vi "Data_Element_Retrieved.vi"(9 "文件名":string, 10 "路径":path=path "F:/report", 11 "Cluster67":T1) -> ()   [LabVIEW 2019]
uses:
  Cluster67.ctl
  <vilib>/Utility/NIReport.llb/Report Type.ctl
  <vilib>/addons/_office/word.llb/Word Find & Replace (str).vi
  <vilib>/Utility/NIReport.llb/NI_ReportGenerationCore.lvlib
  <vilib>/Utility/NIReport.llb/NI_report.lvclass
  <vilib>/addons/_office/NI_ReportGenerationToolkit.lvlib
  <vilib>/Utility/NIReport.llb/Word/NI_Word.lvclass
  TEST.lvclass
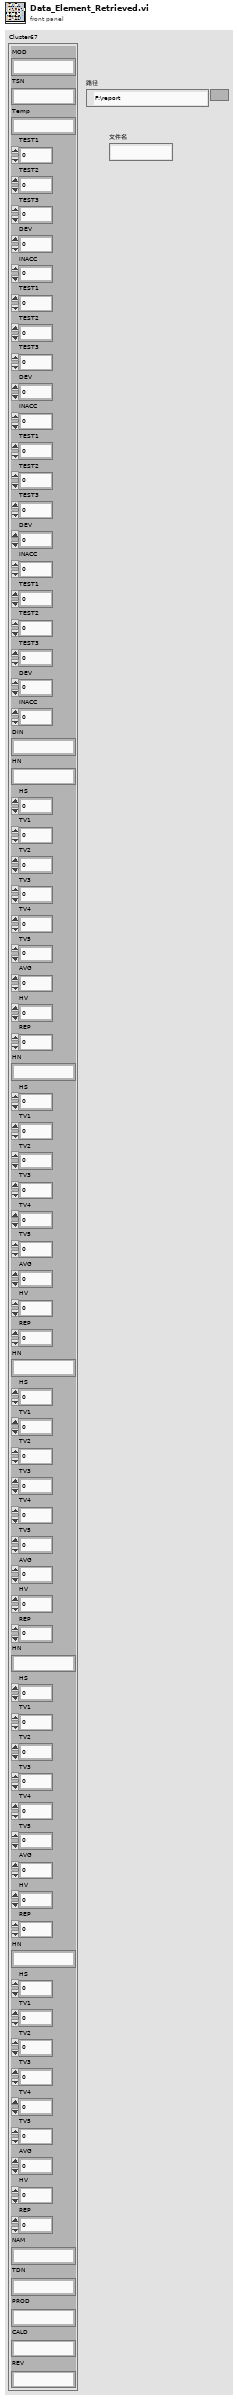
[diagram p1: front panel]
types:
  T1 = typedef "TEST.lvclass/Cluster67.ctl" = cluster{"MOD":string, "TSN":string, "Temp":string, "TEST1":sgl, "TEST2":sgl, "TEST3":sgl, "DEV":sgl, "INACC":sgl, "TEST1":sgl, "TEST2":sgl, "TEST3":sgl, "DEV":sgl, "INACC":sgl, "TEST1":sgl, "TEST2":sgl, "TEST3":sgl, "DEV":sgl, "INACC":sgl, "TEST1":sgl, "TEST2":sgl, "TEST3":sgl, "DEV":sgl, "INACC":sgl, "DIN":string, "HN":string, "HS":sgl, "TV1":sgl, "TV2":sgl, "TV3":sgl, "TV4":sgl, "TV5":sgl, "AVG":sgl, "HV":sgl, "REP":sgl, "HN":string, "HS":sgl, "TV1":sgl, "TV2":sgl, "TV3":sgl, "TV4":sgl, "TV5":sgl, "AVG":sgl, "HV":sgl, "REP":sgl, "HN":string, "HS":sgl, "TV1":sgl, "TV2":sgl, "TV3":sgl, "TV4":sgl, "TV5":sgl, "AVG":sgl, "HV":sgl, "REP":sgl, "HN":string, "HS":sgl, "TV1":sgl, "TV2":sgl, "TV3":sgl, "TV4":sgl, "TV5":sgl, "AVG":sgl, "HV":sgl, "REP":sgl, "HN":string, "HS":sgl, "TV1":sgl, "TV2":sgl, "TV3":sgl, "TV4":sgl, "TV5":sgl, "AVG":sgl, "HV":sgl, "REP":sgl, "NAM":string, "TDN":string, "PROD":string, "CALD":string, "REV":string}
  T2 = typedef "NI_ReportGenerationCore.lvlib/Report Type.ctl" = enum16{"HTML", "Word", "Excel"}
  T3 = enum16{"maximized", "minimized", "normal", "no change"}
  T4 = typedef "TEST.lvclass/Test_data.ctl" = cluster{"MODE":string, "TSN":string, "Temp":string, "Test_load_row1":T5, "Test_load_row2":T5, "Test_load_row3":T5, "Test_load_row4":T5, "DIN":string, "Hardness_test_row1":T6, "Hardness_test_row2":T6, "Hardness_test_row3":T6, "Hardness_test_row4":T6, "Hardness_test_row5":T6}
  T5 = typedef "TEST.lvclass/Test_load.ctl" = cluster{"TEST1":sgl, "TEST2":sgl, "TEST3":sgl, "DEV":sgl, "INACC":sgl}
  T6 = typedef "TEST.lvclass/Hardness_test.ctl" = cluster{"HN":string, "HS":sgl, "TV1":sgl, "TV2":sgl, "TV3":sgl, "TV4":sgl, "TV5":sgl, "AVG":sgl, "HV":sgl, "REP":sgl}
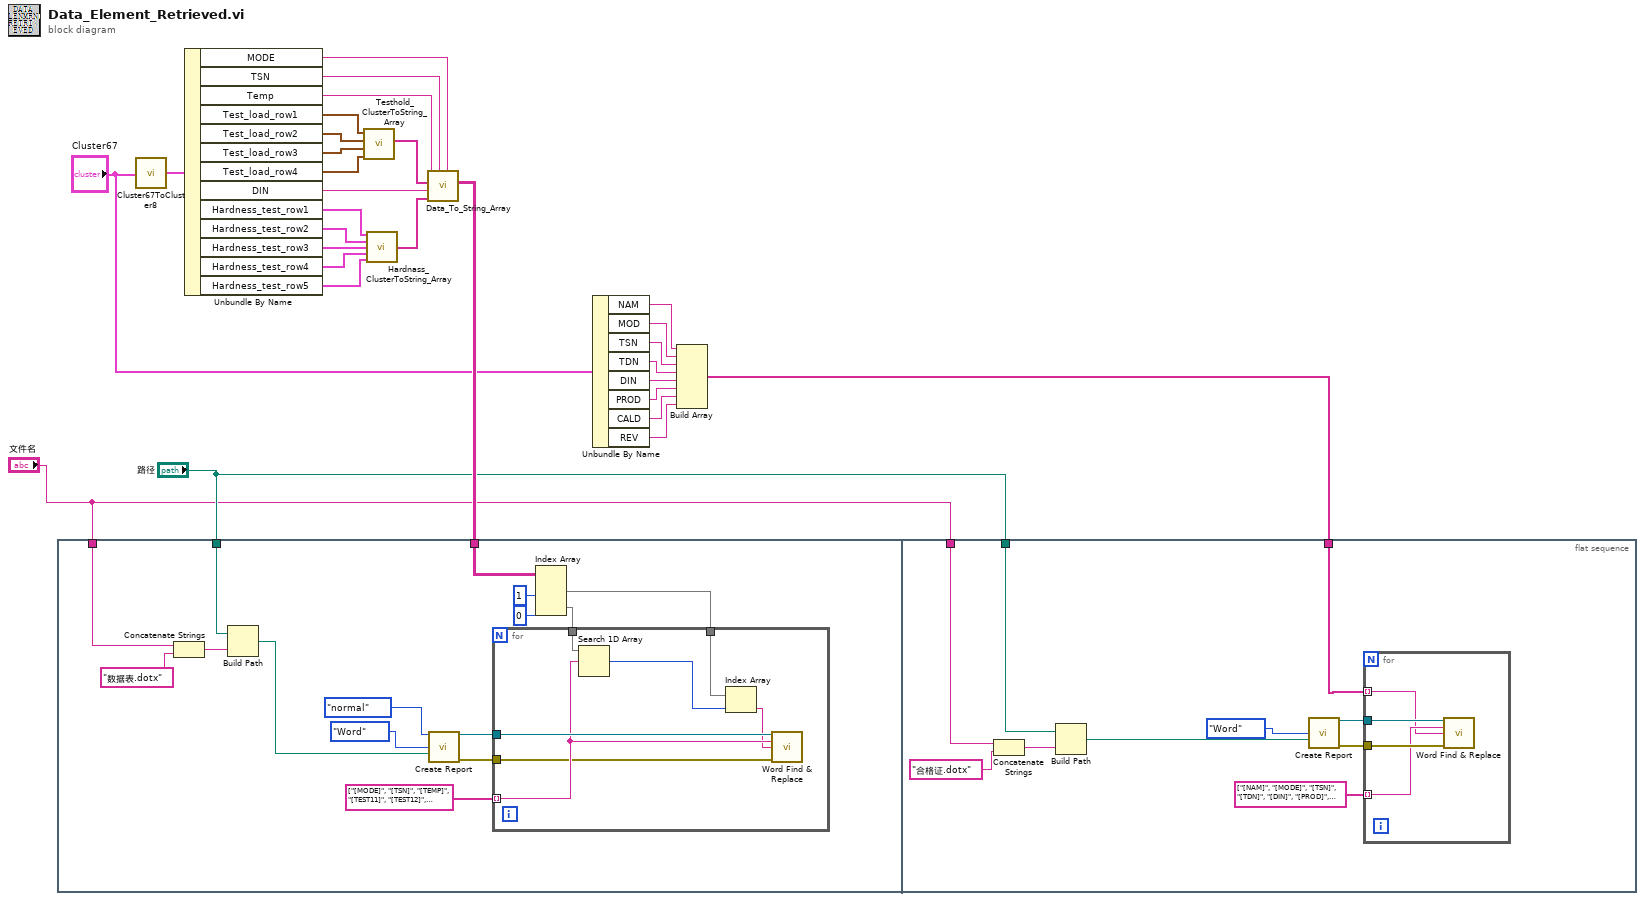
[diagram p0: block diagram]
diagram:
  n1 = flat-sequence {
    tunnel: w13 -> [w35]
    tunnel: "路径" -> [w39]
    tunnel: "文件名" -> [w36]
    tunnel: "路径" -> [w54]
    tunnel: "文件名" -> [w53]
    tunnel: w2 -> [w52]
    frame #0 {
      n2 = Concatenate Strings(w36, "数据表.dotx" ("字符串")) -> (w38:string)
      n3 = Build Path(base path=w39, name or relative path=w38) -> (appended path=w40:path)
      n4 = call <vilib>:"Create Report.vi"("window state (normal)"=T3."normal", "report type"=Report_Type."Word", "template (empty)"=w40) -> ("report out"=w42:refnum<class "NI_report.lvclass">, "error out"=w41:errorcluster)  [unwired: 11 in]
      n5 = Index Array(array=w35, index (col) #1=1 ("禁用的索引 (列)"), index (col) #2=0 ("索引 (列)")) -> (element #1=w31:string[], element #2=w32:string[])  [unwired: 2 in]
      n6 = for {
        tunnel: string[] ["[MODE]", "[TSN]", "[TEMP]", "[TEST11]", "[TEST12]", "[TEST13]", "[DEV1]", "[INACC1]", "[TEST21]", "[TEST22]", "[TEST23]", "[DEV2]", "[INACC2]", "[TEST31]", "[TEST32]", "[TEST33]", "[DEV3]", "[INACC3]", "[TEST41]", "[TEST42]", "[TEST43]", "[DEV4]", "[INACC4]", "[DIN]", "[HN1]", "[HS1]", "[TV11]", "[TV12]", "[TV13]", "[TV14]", "[TV15]", "[AVG1]", "[HV1]", "[REP1]", "[HN2]", "[HS2]", "[TV21]", "[TV22]", "[TV23]", "[TV24]", "[TV25]", "[AVG2]", "[HV2]", "[REP2]", "[HN3]", "[HS3]", "[TV31]", "[TV32]", "[TV33]", "[TV34]", "[TV35]", "[AVG3]", "[HV3]", "[REP3]", "[HN4]", "[HS4]", "[TV41]", "[TV42]", "[TV43]", "[TV44]", "[TV45]", "[AVG4]", "[HV4]", "[REP4]", "[HN5]", "[HS5]", "[TV51]", "[TV52]", "[TV53]", "[TV54]", "[TV55]", "[AVG5]", "[HV5]", "[REP5]"] ("待写入项") -> [w50] mode=indexing
        tunnel: w42 -> [w51]
        tunnel: w41 -> [w49]
        tunnel: w32 -> [w48]
        tunnel: w31 -> [w47]
        n7 = Search 1D Array(1D array=w48, element=w50) -> (index of element=w46:i32)  [unwired: 1 in]
        n8 = Index Array(array=w47, index=w46) -> (element=w45:string)
        n9 = call-poly <vilib>:"Word Find & Replace.vi"("report in"=w51, "find what?"=w50, "replace with"=w45, "error in (no error)"=w49) -> ()  [unwired: 9 in, 3 out]
      }
    }
    frame #1 {
      n10 = Concatenate Strings(w53, "合格证.dotx" ("名称或相对路径")) -> (w57:string)
      n11 = Build Path(base path=w54, name or relative path=w57) -> (appended path=w61:path)
      n12 = call <vilib>:"Create Report.vi"("report type"=Report_Type."Word", "template (empty)"=w61) -> ("report out"=w59:refnum<class "NI_report.lvclass">, "error out"=w58:errorcluster)  [unwired: 12 in]
      n13 = for {
        tunnel: w59 -> [w65]
        tunnel: w58 -> [w64]
        tunnel: string[] ["[NAM]", "[MODE]", "[TSN]", "[TDN]", "[DIN]", "[PROD]", "[CALD]", "[REV]"] ("待写入项 2") -> [w63] mode=indexing
        tunnel: w52 -> [w62] mode=indexing
        n14 = call-poly <vilib>:"Word Find & Replace.vi"("report in"=w65, "find what?"=w63, "replace with"=w62, "error in (no error)"=w64) -> ()  [unwired: 9 in, 3 out]
      }
    }
  }
  n15 = call "Cluster67ToCluster8.vi"("Cluster67"="Cluster67") -> ("Cluster8"=w29:T4)  [unwired: 1 in]
  n16 = Unbundle By Name(w29) -> ("MODE"=w25:string, "TSN"=w26:string, "Temp"=w27:string, "Test_load_row1"=w18:T5, "Test_load_row2"=w17:T5, "Test_load_row3"=w16:T5, "Test_load_row4"=w15:T5, "DIN"=w28:string, "Hardness_test_row1"=w24:T6, "Hardness_test_row2"=w23:T6, "Hardness_test_row3"=w22:T6, "Hardness_test_row4"=w21:T6, "Hardness_test_row5"=w20:T6)
  n17 = call "Testhold_ClusterToString_Array.vi"("SLG_Cluster4"=w15, "SLG_Cluster3"=w16, "SLG_Cluster2"=w17, "SLG_Cluster"=w18) -> ("String_Array"=w14:string[])  [unwired: 7 in]
  n18 = call "Hardnass_ClusterToString_Array.vi"("Hardness_test"=w24, "Hardness_test 2"=w23, "Hardness_test 3"=w22, "Hardness_test 4"=w21, "Hardness_test 5"=w20) -> ("StringArray"=w19:string[])  [unwired: 10 in]
  n19 = call "Data_To_String_Array.vi"("MODE"=w25, "TSN"=w26, "Hardness_string"=w19, "DIN"=w28, "Test_load_string"=w14, "TEMP"=w27) -> ("String_Array"=w13:string[][])  [unwired: 5 in]
  n20 = Unbundle By Name("Cluster67") -> ("NAM"=w10:string, "MOD"=w9:string, "TSN"=w8:string, "TDN"=w7:string, "DIN"=w6:string, "PROD"=w5:string, "CALD"=w4:string, "REV"=w3:string)
  n21 = Build Array(w10, w9, w8, w7, w6, w5, w4, w3) -> (w2:string[])
